vi "Send Update Fan Status.vi"(5 "Update Msg Object":refnum<class "Update Fan Status Msg.lvclass">, 7 "Message Priority (Normal)":T2=enum."Normal", 8 "error in (no error)":errorcluster, 9 "Fan B":T1, 10 "Fan A":T1, 11 "Message Enqueuer":refnum<class "Message Enqueuer.lvclass">) -> (0 "error out":errorcluster)   [LabVIEW 2025, in "Dual Fan.lvlib" / "Update Fan Status Msg.lvclass"]
doc: "This VI sends the message to an actor."
uses:
  Update Fan Status Msg.lvclass
  <vilib>/ActorFramework/Message Enqueuer/Message Enqueuer.lvclass
  <vilib>/ActorFramework/Message Enqueuer/Message Priority.ctl
  Dual Fan/Fan Info.ctl
  C:/Program Files/National Instruments/LabVIEW 2025/vi.lib/ActorFramework/Message/Message.lvclass
  Update Fan Status Msg.lvclass/Update Fan Status Msg.ctl
  <vilib>/ActorFramework/Message Enqueuer/Message Enqueuer.lvclass/Message Enqueuer.ctl
  <vilib>/ActorFramework/Message Priority Queue/Priority Enqueue.vi
  Dual Fan/Dual Fan.lvclass
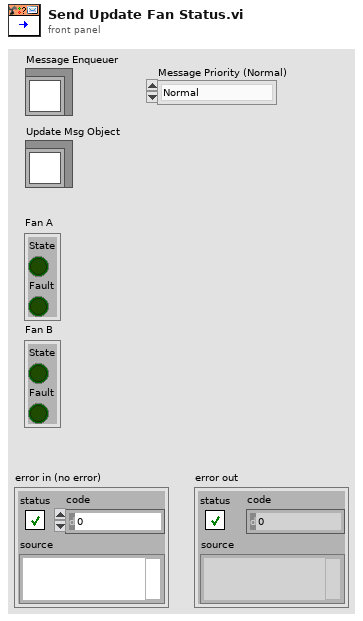
[diagram p1: front panel]
types:
  T1 = typedef "Dual Fan.lvlib/Dual Fan.lvclass/Fan Info.ctl" = cluster{"State":bool, "Fault":bool}
  T2 = typedef "Actor Framework.lvlib/Message Enqueuer.lvclass/Message Priority.ctl" = enum16{"Low", "Normal", "High"}
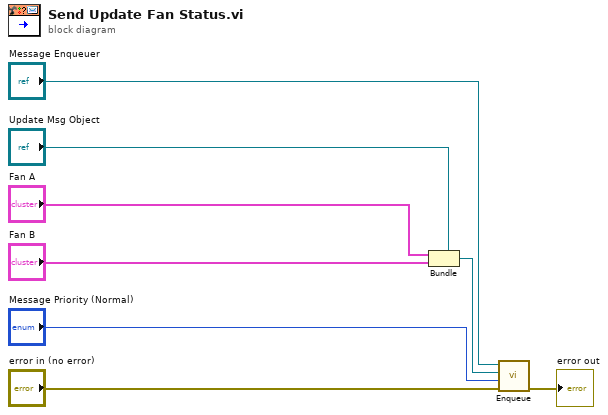
[diagram p0: block diagram]
diagram:
  n1 = Bundle(cluster="Update Msg Object", "Fan A", "Fan B") -> (w5:refnum<class "Update Fan Status Msg.lvclass">)
  n2 = call <vilib>:"Enqueue.vi"("error in (no error)"="error in (no error)", "Message Priority (Normal)"="Message Priority (Normal)", "Message"=w5, "Message Enqueuer in"="Message Enqueuer") -> ("error out"=→"error out":errorcluster)  [unwired: 6 in, 1 out]
